vi "AutoScore.vi"() -> ()   [LabVIEW 2019]
panel:
  in  "ShooterSpeed":dbl
  in  "LimelightDistance":bool
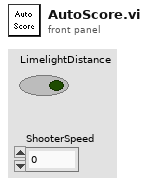
[diagram p1: front panel]
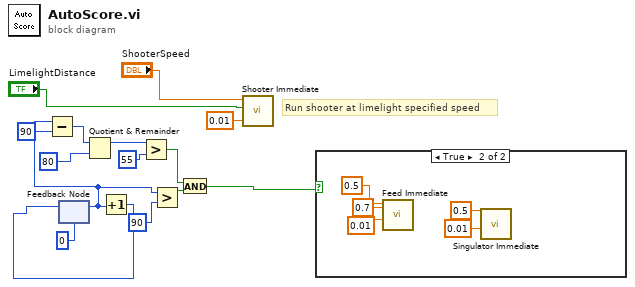
[diagram p0: block diagram]
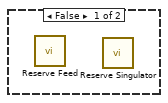
[diagram p2: hidden frame]
diagram:
  # "Run shooter at limelight specified speed"
  n1 = feedback #1(0) -> (w6:i32)
  n2 = Subtract(x=w6, y=90) -> (x-y=w5:i32)
  n3 = Quotient & Remainder(x=w5, y=80) -> (x-y*floor(x/y)=w13:i32)  [unwired: 1 out]
  n4 = Increment(x=w6) -> (x+1=w3:i32)
  n5 = feedback-in #1(w3) -> ()
  n6 = Greater?(x=w13, y=55) -> (0:w10:bool)
  n7 = Greater?(x=w6, y=90) -> (0:w9:bool)
  n8 = And(x=w10, y=w9) -> (x .and. y?=w4:bool)
  n9 = call "Shooter Immediate.vi"("Deadband Value"=0.01, "LimeLightDistance?"="LimelightDistance", "Setpoint"="ShooterSpeed") -> ()  [unwired: 8 in, 1 out]
  n10 = case shown="True" w4 {
    frame False {
      n11 = call "Reserve Feed.vi"() -> ()  [unwired: 11 in, 1 out]
      n12 = call "Reserve Singulator.vi"() -> ()  [unwired: 11 in, 1 out]
    }
    frame True {
      n13 = call "Feed Immediate.vi"("Deadband Value"=0.01, "Upper Setpoint"=0.7, "Lower Setpoint"=0.5) -> ()  [unwired: 8 in, 1 out]
      n14 = call "Singulator Immediate.vi"("Deadband"=0.01, "Setpoint"=0.5) -> ()  [unwired: 9 in, 1 out]
    }
  }
